vi "Read Data.vi"(8 "OLD":i32, 9 "DataBuf":u32[](array[numeric]), 10 "GateNum":i32, 11 "handle":i32) -> (0 "OLD out":i32, 1 "DataBuf out":u32[](array[numeric]), 2 "GateNum out":i32, 3 "handle out":i32, 5 "function return":u32)   [LabVIEW 2022 SP3]
doc: "DWORD H11890API __stdcall H11890ReadData(HANDLE handle,DWORD *GateNum,DWORD *DataBuf,BOOL *OLD);"
uses:
  H11890api.dll
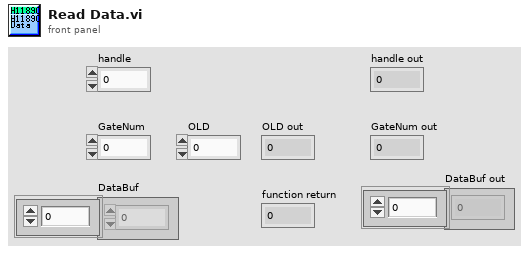
[diagram p1: front panel]
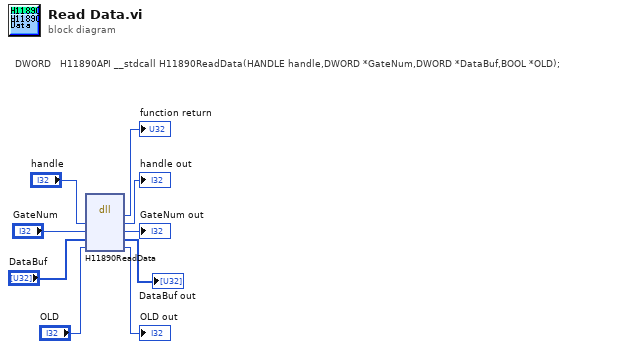
[diagram p0: block diagram]
diagram:
  # "DWORD\t\t\tH11890API __stdcall H11890ReadData(HANDLE handle,DWORD *GateNum,DWORD *DataBuf,BOOL *OLD);"
  n1 = dll-call lib="H:/.shortcut-targets-by-id/1riZacJd_1_jmKfGgrjDuP7KcecvMS3i2/Xiao research group/Programs/LabviewControlPrograms/scanner_stepper_and_mapping/PMT_mapping/H11890api.dll" fn="H11890ReadData"("handle"="handle", "GateNum"="GateNum", "DataBuf"="DataBuf", "OLD"="OLD") -> ("Return"=→"function return":u32, "handle"=→"handle out":i32, "GateNum"=→"GateNum out":i32, "DataBuf"=→"DataBuf out":u32[], "OLD"=→"OLD out":i32)  [unwired: 3 in, 2 out]
